vi "Read Caster Angle.vi"(8 "error in (no error)":errorcluster, 11 "caster wheel in":refnum<class "NI_Robotics_Caster Wheel.lvclass">) -> (0 "error out":errorcluster, 1 "failed":bool, 2 "caster angle (rad)":dbl, 3 "caster wheel out":refnum<class "NI_Robotics_Caster Wheel.lvclass">)   [LabVIEW 2017, in "NI_Robotics_Caster Wheel.lvclass"]
uses:
  <vilib>/robotics/Steering/Caster Wheel/NI_Robotics_Caster Wheel.lvclass
  <vilib>/robotics/Steering/Caster Wheel/NI_Robotics_Caster Wheel.lvclass/NI_Robotics_Caster Wheel.ctl
  <vilib>/robotics/Actuation/Motor Communication/Check if Valid.vi
  <vilib>/robotics/Utilities/Generate Error.vi
  <vilib>/robotics/Actuation/Motor Communication/NI_Robotics_Motor Communication.lvclass
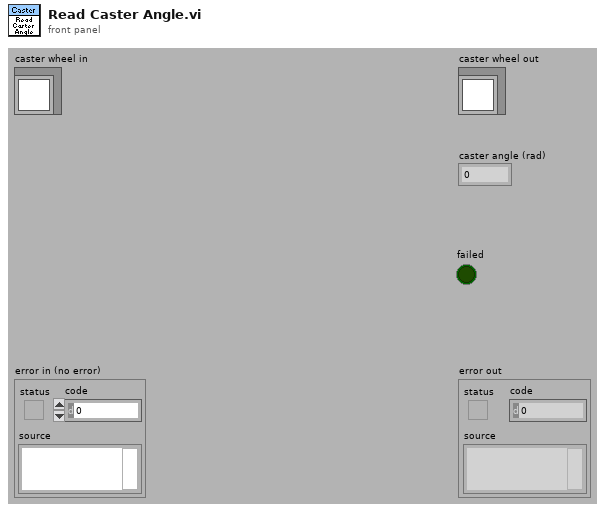
[diagram p1: front panel]
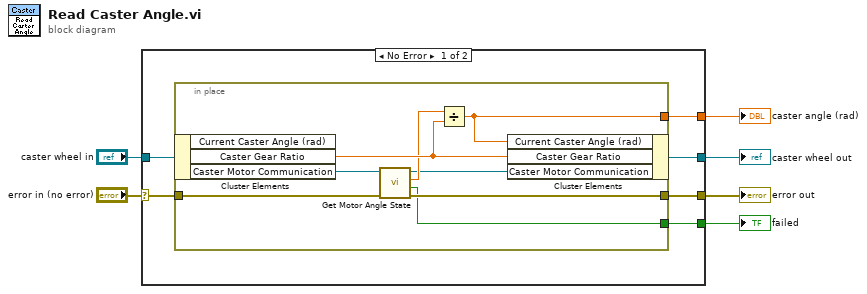
[diagram p0: block diagram]
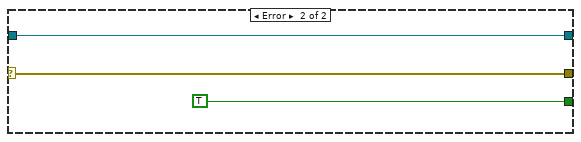
[diagram p2: hidden frame]
diagram:
  n1 = case shown="No Error" "error in (no error)" {
    selector: "error in (no error)" -> [w11 w23]
    tunnel: "caster wheel in" -> [w12 w22]
    tunnel: [w9 w23] -> w4
    tunnel: [w10 w22] -> w3
    tunnel: [w7 TRUE] -> w2
    tunnel: [w8 _] -> w1
    frame No Error {
      n2 = in-place {
        in-place-border: w11 -> [w16]
        in-place-border: [w15] -> w9
        in-place-border: [w19] -> w8
        in-place-border: [w13] -> w7
        n3 = in-place-cluster #1(w12) -> ("Caster Gear Ratio"=w20:dbl, "Caster Motor Communication"=w17:refnum<class "NI_Robotics_Motor Communication.lvclass">)  [unwired: 1 out]
        n4 = call <vilib>:"Get Motor Angle State.vi"("error in (no error)"=w16, "motor communication in"=w17) -> ("error out"=w15:errorcluster, "failed?"=w13:bool, "angle"=w18:dbl, "motor communication out"=w14:refnum<class "NI_Robotics_Motor Communication.lvclass">)  [unwired: 6 in]
        n5 = Divide(x=w18, y=w20) -> (x/y=w19:dbl)
        n6 = in-place-cluster #1("Current Caster Angle (rad)"=w19, "Caster Gear Ratio"=w20, "Caster Motor Communication"=w14) -> (w10:refnum<class "NI_Robotics_Caster Wheel.lvclass">)
      }
    }
    frame Error {
    }
  }
  "error out" <- w4
  "caster wheel out" <- w3
  "caster angle (rad)" <- w1
  "failed" <- w2
